vi "LoadPlugin.vi"(8 "error in (no error)":errorcluster, 9 "Module Name":string, 10 "INI File Path":path, 11 "Module ID":i32) -> (0 "error out":errorcluster, 1 "Module Name out":string, 2 "INI File Path out":path, 3 "Module ID out":i32)   [LabVIEW 2018, in "Test.lvclass"]
uses:
  Test.lvclass
  <vilib>/Utility/error.llb/Error Cluster From Error Code.vi
  <vilib>/ErrorRing/Error Ring.xnode
  Sync/SyncPlugins/SyncPluginBase/SyncPluginBase.lvclass
  FGen/FgenPlugins/FgenPluginBaseClass/FgenPluginsBase.lvclass
  Scope/ScopeModule/ScopeModule.lvlib
  Digitizer/DigitizerPlugins/DigitizerBaseClass/DigitizerBase.lvclass
  Sensor/SensorModule/SensorModule.lvlib
  Analysis/AnalysisPlugins/AnalysisPluginBaseClass/AnalysisPluginsBase.lvclass
  AcPwr/AcPwrModule/AcPwrModule.lvlib
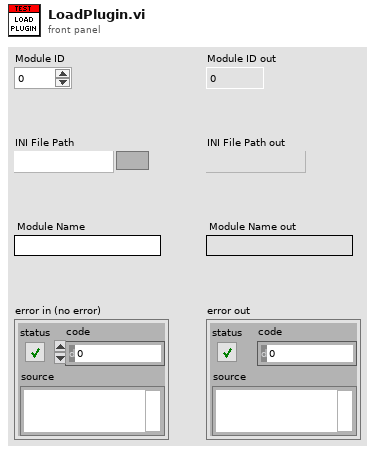
[diagram p1: front panel]
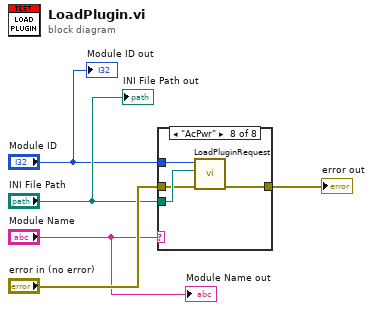
[diagram p0: block diagram]
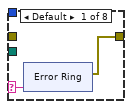
[diagram p2: hidden frame]
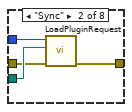
[diagram p3: hidden frame]
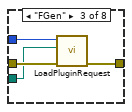
[diagram p4: hidden frame]
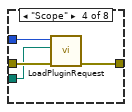
[diagram p5: hidden frame]
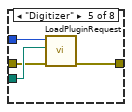
[diagram p6: hidden frame]
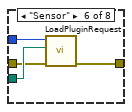
[diagram p7: hidden frame]
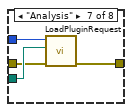
[diagram p8: hidden frame]
diagram:
  n1 = case shown="\"AcPwr\"" "Module Name" {
    selector: "Module Name" -> [w7 _ _ _ _ _ _ _]
    tunnel: "Module ID" -> [_ w18 w19 w23 w30 w34 w38 w42]
    tunnel: "INI File Path" -> [_ w17 w20 w24 w29 w33 w37 w41]
    tunnel: "error in (no error)" -> [_ w16 w22 w25 w28 w32 w36 w40]
    tunnel: [w6 w15 w21 w26 w27 w31 w35 w39] -> w3
    frame Default {
      n2 = xnode "Error Ring"("parameter 0"=w7) -> ("error out"=w6:errorcluster)
    }
    frame "Sync" {
      n3 = call "LoadPluginRequest.vi"("error in (no error)"=w16, "PathToPluginINI"=w17, "ModuleID"=w18) -> ("error out"=w15:errorcluster)  [unwired: 8 in]
    }
    frame "FGen" {
      n4 = call "LoadPluginRequest.vi"("error in (no error)"=w22, "PathToPluginINI"=w20, "ModuleID"=w19) -> ("error out"=w21:errorcluster)  [unwired: 8 in]
    }
    frame "Scope" {
      n5 = call "LoadPluginRequest.vi"("error in (no error)"=w25, "PathToPluginINI"=w24, "ModuleID"=w23) -> ("error out"=w26:errorcluster)  [unwired: 8 in]
    }
    frame "Digitizer" {
      n6 = call "LoadPluginRequest.vi"("error in (no error)"=w28, "PathToPluginINI"=w29, "ModuleID"=w30) -> ("error out"=w27:errorcluster)  [unwired: 8 in]
    }
    frame "Sensor" {
      n7 = call "LoadPluginRequest.vi"("error in (no error)"=w32, "PathToPluginINI"=w33, "ModuleID"=w34) -> ("error out"=w31:errorcluster)  [unwired: 8 in]
    }
    frame "Analysis" {
      n8 = call "LoadPluginRequest.vi"("error in (no error)"=w36, "PathToPluginINI"=w37, "ModuleID"=w38) -> ("error out"=w35:errorcluster)  [unwired: 8 in]
    }
    frame "AcPwr" {
      n9 = call "LoadPluginRequest.vi"("error in (no error)"=w40, "PathToPluginINI"=w41, "ModuleID"=w42) -> ("error out"=w39:errorcluster)  [unwired: 8 in]
    }
  }
  "error out" <- w3
  "Module ID out" <- "Module ID"
  "INI File Path out" <- "INI File Path"
  "Module Name out" <- "Module Name"
